vi "String_to_Pos_array.vi"(2 "Channel values":string[][](array[string]), 3 "Channel names":string[](array[string])) -> (0 "Positions":dbl[][](array[numeric]) format="%.2f", 1 "No of Inst":i32)   [LabVIEW 2010]
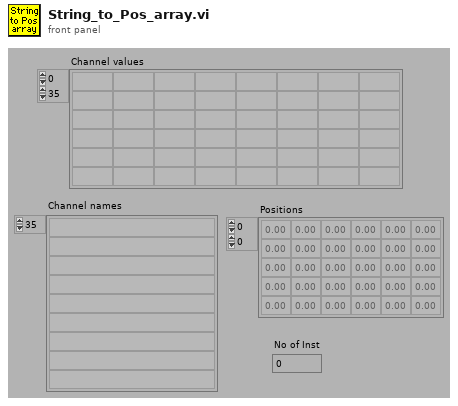
[diagram p1: front panel]
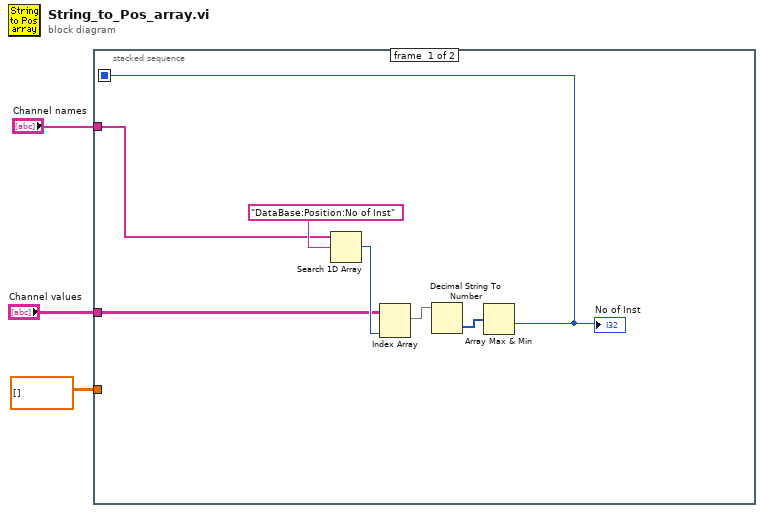
[diagram p0: block diagram]
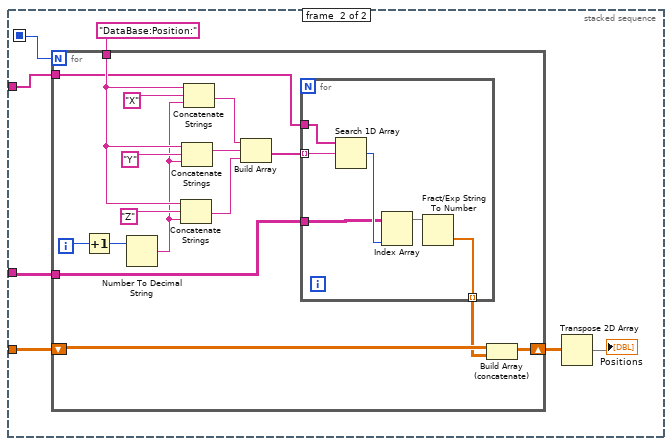
[diagram p2: hidden frame]
diagram:
  n1 = stacked-sequence {
    seq-local: [w4 _] -> [_ w17]
    tunnel: "Channel names" -> [w9 w15]
    tunnel: "Channel values" -> [w7 w14]
    tunnel: dbl[][] [] -> [_ w11]
    frame #0 {
      n2 = Search 1D Array(1D array=w9, element="DataBase:Position:No of Inst") -> (index of element=w8:i32)  [unwired: 1 out]
      n3 = Index Array(array=w7, index (col)=w8) -> (element=w6:string[])  [unwired: 1 in]
      n4 = Decimal String To Number(string=w6) -> (number=w5:i32[])  [unwired: 3 out]
      n5 = Array Max & Min(array=w5) -> (min value=w4:i32)  [unwired: 3 out]
      "No of Inst" <- w4
    }
    frame #1 {
      n6 = for {
        N: w17 -> [_]
        tunnel: "DataBase:Position:" -> [w28]
        tunnel: w15 -> [w23]
        tunnel: w14 -> [w21]
        shift-right: [w18] -> w13
        shift-left: w11 -> [w20]
        i -> [w31]
        n7 = Increment(x=w31) -> (x+1=w32:i32)
        n8 = Number To Decimal String(number=w32) -> (decimal integer string=w27:string)  [unwired: 1 out]
        n9 = Concatenate Strings(w28, "Z", w27) -> (w24:string)
        n10 = Concatenate Strings(w28, "Y", w27) -> (w25:string)
        n11 = Concatenate Strings(w28, "X", w27) -> (w26:string)
        n12 = Build Array(w26, w25, w24) -> (w22:string[])
        n13 = for {
          tunnel: w23 -> [w39]
          tunnel: w22 -> [w38] mode=indexing
          tunnel: w21 -> [w36]
          tunnel: [w34] -> w19 mode=indexing
          n14 = Search 1D Array(1D array=w39, element=w38) -> (index of element=w37:i32)  [unwired: 1 out]
          n15 = Index Array(array=w36, index (col)=w37) -> (element=w35:string[])  [unwired: 1 in]
          n16 = Fract/Exp String To Number(string=w35) -> (number=w34:dbl[])  [unwired: 4 out]
        }
        n17 = Build Array (concatenate)(w20, w19) -> (w18:dbl[][])
      }
      n18 = Transpose 2D Array(2D array=w13) -> (transposed array=→"Positions":dbl[][])
    }
  }
